vi "Update PhXP Parameters.vi"(8 "error in (no error)":errorcluster, 11 "VI in":refnum<vi>) -> (0 "error out":errorcluster, 2 "tau*":dbl[unit], 3 "f0":dbl[unit])   [LabVIEW 2019]
uses:
  Phasor Explorer Phasor Parameters.ctl
  Phasor Calculation Type.ctl
  SEPL Type.ctl
  Phasor Explorer Gate Parameters.ctl
  Gate Type.ctl
  SEPXP Gate Parameter to Adjust.ctl
  Phasor Explorer Decay Parameters.ctl
  IRF Model.ctl
  Phasor Explorer Display Parameters.ctl
  Type of Series.ctl
  Phasor Explorer Detector Parameters.ctl
panel:
  in  "Phasor Explorer Detector Parameters":T1={"Frames/Image"=0, "Gates/Frame"=1, "Bits/Frame"=1, "Multiplicity"=0, "Incident Signal"=0.0, "Poisson Signal"=FALSE} {"Frames/Image" min=1; "Multiplicity" min=0; "Bits/Frame" min=1; "Gates/Frame" min=1}
  in  "Edit User-defined Gate":bool
  in  "Phasor Explorer Display Parameters":T2={"# Points"=1, "Ramp Type"=enum."Linear", "Type of Series"=enum."1-Exp Decays", "Min tau"=0.0, "Max tau"=0.0, "Include 0"=FALSE, "Include Infinity"=FALSE} {"Min tau" min=0.0; "Max tau" min=0.0; "# Points" min=1 step=1}
  in  "Phasor Explorer Decay & IRF Parameters":T4 {"Lifetime" min=0.0; "IRF Period" min=0.0}
  in  "Gate Parameter to Adjust":T6 caption="Parameter to adjust"
  in  "Phasor Explorer Gate Parameters":T7={"First Gate Start"=0.0, "Use Gate Center"=FALSE, "Gate Width"=0.0, "Gate Step"=0.0, "# Gates"=1.0, "Gate Type"=enum."Square", "Edge Width"=0.0, "Top Slope"=0.0, "Reversed Sawtooth?"=FALSE, "Analytical Computation"=FALSE, "Integration"=enum."Item 0", "Tolerance"=1.0, "# Steps"=1.0, "Type of User-defined Function"=enum."Gate", "Use Gate Step"=FALSE} {"# Steps" min=0.0; "Tolerance" min=0.0; "Top Slope" min=0.0; "Edge Width" min=0.0; "Gate Step" min=0.0; "# Gates" min=1.0 step=1.0; "Gate Width" min=0.0}
  in  "Phasor Explorer Phasor Parameters":T9={"Harmonic frequency"=0.0, "Use f* = 1/D Frequency"=FALSE, "Calibrated Phasor"=FALSE, "Calibration Lifetime"=1e-09, "Phasor Calculation"=enum."Direct Sum", "SEPL Type"=enum."UC", "# Gates"=1.0, "Square Gate Width"=1e-09, "Show Ticks"=FALSE} {"Square Gate Width" min=0.0; "# Gates" min=0.0; "Calibration Lifetime" min=0.0; "Harmonic frequency" min=0.0}
  in  "Match Laser Period":bool
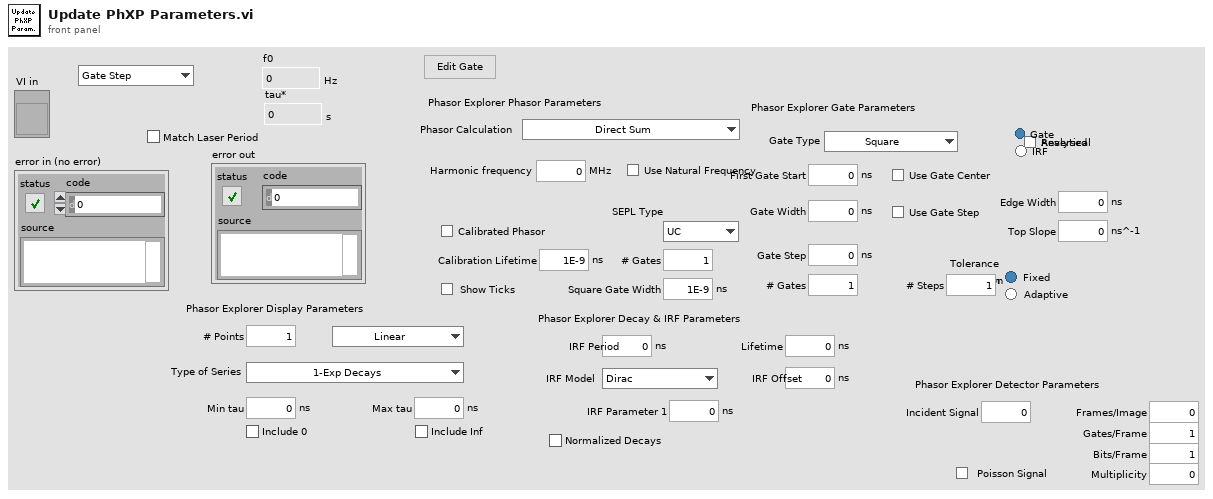
[diagram p1: front panel]
types:
  T1 = typedef "Phasor Explorer Detector Parameters.ctl" = cluster{"Frames/Image":i32, "Gates/Frame":i32, "Bits/Frame":i32, "Multiplicity":i32, "Incident Signal":dbl, "Poisson Signal":bool}
  T2 = typedef "Phasor Explorer Display Parameters.ctl" = cluster{"# Points":i32, "Ramp Type":enum16{"Linear", "Logarithmic"}, "Type of Series":T3, "Min tau":dbl[unit], "Max tau":dbl[unit], "Include 0":bool, "Include Infinity":bool}
  T3 = typedef "Type of Series.ctl" = enum16{"1-Exp Decays", "Linear Combination of 1-Exp"}
  T4 = typedef "Phasor Explorer Decay Parameters.ctl" = cluster{"Lifetime":dbl[unit], "IRF Offset":dbl[unit], "IRF Period":dbl[unit], "Normalized Decays":bool, "IRF Model":T5, "IRF Parameter 1":dbl[unit]}
  T5 = typedef "IRF Model.ctl" = enum16{"Dirac", "Exponential"}
  T6 = typedef "SEPXP Gate Parameter to Adjust.ctl" = enum16{"Gate Step", "# Gates"}
  T7 = typedef "Phasor Explorer Gate Parameters.ctl" = cluster{"First Gate Start":dbl[unit], "Use Gate Center":bool, "Gate Width":dbl[unit], "Gate Step":dbl[unit], "# Gates":dbl, "Gate Type":T8, "Edge Width":dbl[unit], "Top Slope":dbl[unit], "Reversed Sawtooth?":bool, "Analytical Computation":bool, "Integration":enum32{"Item 0", "Item 1"}, "Tolerance":dbl, "# Steps":dbl, "Type of User-defined Function":enum32{"Gate", "IRF"}, "Use Gate Step":bool}
  T8 = typedef "Gate Type.ctl" = enum16{"Square", "Finite Edge Square", "Finite Edge, Tilted Top Square", "Triangle", "Sawtooth", "User-defined"}
  T9 = typedef "Phasor Explorer Phasor Parameters.ctl" = cluster{"Harmonic frequency":dbl[unit], "Use f* = 1/D Frequency":bool, "Calibrated Phasor":bool, "Calibration Lifetime":dbl[unit], "Phasor Calculation":T10, "SEPL Type":T11, "# Gates":dbl, "Square Gate Width":dbl[unit], "Show Ticks":bool}
  T10 = typedef "Phasor Calculation Type.ctl" = enum16{"Direct Sum", "Analytical Formula"}
  T11 = typedef "SEPL Type.ctl" = enum16{"UC", "L_N", "L_N[W]"}
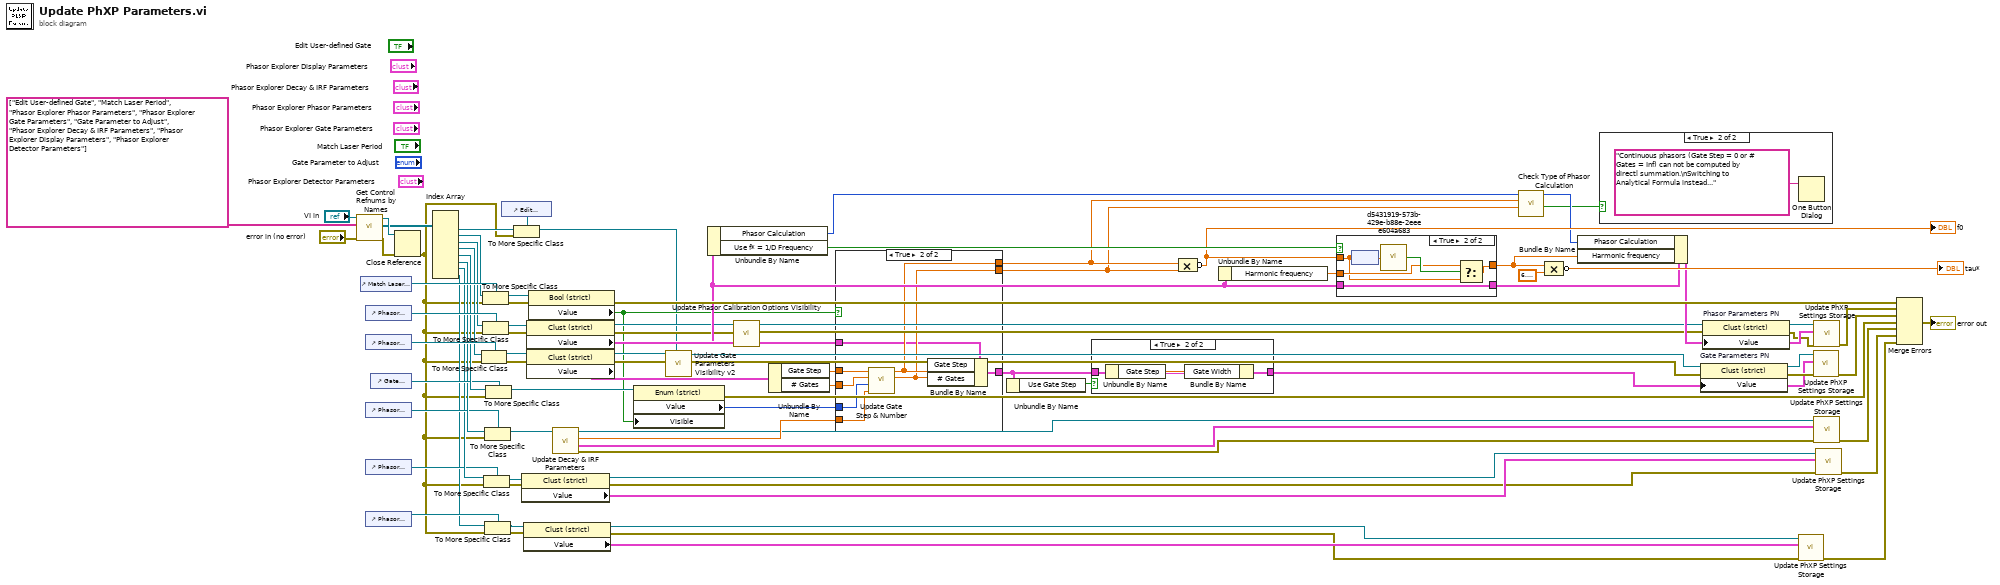
[diagram p0: block diagram]
diagram:
  n1 = call "Get Control Refnums by Names.vi"("error in"="error in (no error)", "Control Labels"=string[] ["Edit User-defined Gate", "Match Laser Period", "Phasor Explorer Phasor Parameters", "Phasor Explorer Gate Parameters", "Gate Parameter to Adjust", "Phasor Explorer Decay & IRF Parameters", "Phasor Explorer Display Parameters", "Phasor Explorer Detector Parameters"], "VI  Ref"="VI in") -> ("error out"=w18:errorcluster, "Ctl Refnums"=w84:refnum<vi>[], "VI  Ref (out)"=w85:refnum<vi>)  [unwired: 5 in, 1 out]
  n2 = control-ref of="Match Laser Period"() -> (w77:refnum<vi>)
  n3 = control-ref of="Phasor Explorer Phasor Parameters"() -> (w80:refnum<vi>)
  n4 = control-ref of="Phasor Explorer Gate Parameters"() -> (w79:refnum<vi>)
  n5 = control-ref of="Phasor Explorer Decay & IRF Parameters"() -> (w58:refnum<vi>)
  n6 = control-ref of="Phasor Explorer Display Parameters"() -> (w39:refnum<vi>)
  n7 = control-ref of="Phasor Explorer Detector Parameters"() -> (w14:refnum<vi>)
  n8 = control-ref of="Gate Parameter to Adjust"() -> (w71:refnum<vi>)
  n9 = Close Reference(reference=w85, error in (no error)=w18) -> (error out=w12:errorcluster)
  n10 = Index Array(array=w84) -> (element #1=w17:refnum<vi>, element #2=w62:refnum<vi>, element #3=w61:refnum<vi>, element #4=w60:refnum<vi>, element #5=w73:refnum<vi>, element #6=w59:refnum<vi>, element #7=w40:refnum<vi>, element #8=w13:refnum<vi>)  [unwired: 8 in]
  n11 = To More Specific Class(target class=w79, reference=w60, error in=w12) -> (specific class reference=w66:refnum<vi>, error out=w65:errorcluster)
  n12 = To More Specific Class(target class=w77, reference=w62, error in=w12) -> (specific class reference=w76:refnum<vi>, error out=w75:errorcluster)
  n13 = To More Specific Class(target class=w80, reference=w61, error in=w12) -> (specific class reference=w68:refnum<vi>, error out=w67:errorcluster)
  n14 = To More Specific Class(target class=w39, reference=w40, error in=w12) -> (specific class reference=w38:refnum<vi>, error out=w37:errorcluster)
  n15 = To More Specific Class(target class=w58, reference=w59, error in=w12) -> (specific class reference=w57:refnum<vi>)  [unwired: 1 out]
  n16 = To More Specific Class(target class=w14, reference=w13, error in=w12) -> (specific class reference=w11:refnum<vi>, error out=w10:errorcluster)
  n17 = To More Specific Class(target class=w71, reference=w73, error in=w12) -> (specific class reference=w72:refnum<vi>)  [unwired: 1 out]
  n18 = control-ref of="Edit User-defined Gate"() -> (w16:refnum<vi>)
  n19 = To More Specific Class(target class=w16, reference=w17, error in=w12) -> (specific class reference=w15:refnum<vi>)  [unwired: 1 out]
  n20 = property class="Clust (strict)"(reference=w38, error in=w37) -> (reference out=w34:refnum<vi>, error out=w32:errorcluster, "Value"=w33:T2)
  n21 = property class="Clust (strict)"(reference=w11, error in=w10) -> (reference out=w9:refnum<vi>, error out=w7:errorcluster, "Value"=w8:T1)
  n22 = property class="Clust (strict)"(reference=w68, error in=w67) -> (reference out=w26:refnum<vi>, error out=w24:errorcluster, "Value"=w47:T9)
  n23 = property class="Clust (strict)"(reference=w66, error in=w65) -> (reference out=w41:refnum<vi>, error out=w22:errorcluster, "Value"=w55:T7)
  n24 = property class="Bool (strict)"(reference=w76, error in=w75) -> (error out=w74:errorcluster, "Value"=w19:bool)  [unwired: 1 out]
  n25 = call "Update Decay & IRF Parameters.vi"("Decay & IRF Parameters Refnum"=w57) -> ("error out"=w29:errorcluster, "Value"=w31:T4, "Laser Period"=w56:dbl[unit], "Decay & IRF Parameters Refnum"=w30:refnum<vi>)  [unwired: 7 in]
  n26 = property class="Enum (strict)"(reference=w72, "Visible"=w19) -> (error out=w69:errorcluster, "Value"=w70:T6)  [unwired: 1 in, 1 out]
  n27 = call "Update Gate Parameters Visibility v2.vi"("Edit User-defined Gate"=w15, "error in (no error)"=w22, "Phasor Explorer Gate Parameters in"=w41) -> ("error out"=w21:errorcluster, "Phasor Explorer Gate Parameters out"=w20:refnum<vi>)  [unwired: 7 in]
  n28 = Unbundle By Name(w47) -> ("Phasor Calculation"=w28:T10, "Use f* = 1/D Frequency"=w83:bool)
  n29 = call "Update Phasor Calibration Options Visibility.vi"("Error In"=w24, "Phasor Explorer Phasor Parameters Refnum in"=w26) -> ("Error Out"=w23:errorcluster, "Phasor Explorer Phasor Parameters Refnum out"=w25:refnum<vi>)  [unwired: 8 in]
  n30 = Unbundle By Name(w55) -> ("Gate Step"=w64:dbl[unit], "# Gates"=w63:dbl)
  n31 = case shown="True" w19 {
    tunnel: w56 -> [_ w93]
    tunnel: [w91 w99] -> w53
    tunnel: [w90 w98] -> w52
    tunnel: w70 -> [_ w97]
    tunnel: w64 -> [w91 w96]
    tunnel: w63 -> [w90 w95]
    tunnel: w55 -> [w89 w94]
    tunnel: [w89 w92] -> w4
    frame False {
    }
    frame True {
      n32 = call "Update Gate Step & Number.vi"("Period"=w93, "Value to Update"=w97, "# Gates in"=w95, "Gate Step in"=w96) -> ("# Gates out"=w98:dbl, "Gate Step out"=w99:dbl[unit])  [unwired: 6 in]
      n33 = Bundle By Name(cluster=w94, "Gate Step"=w99, "# Gates"=w98) -> (w92:T7)
    }
  }
  n34 = Unbundle By Name(w4) -> ("Use Gate Step"=w5:bool)
  n35 = case shown="True" w5 {
    tunnel: w4 -> [w100 w102]
    tunnel: [w100 w101] -> w3
    frame False {
    }
    frame True {
      n36 = Unbundle By Name(w102) -> ("Gate Step"=w103:dbl[unit])
      n37 = Bundle By Name(cluster=w102, "Gate Width"=w103) -> (w101:T7)
    }
  }
  n38 = Compound Arithmetic op=MULTIPLY(w53, w52) -> (invert w48:dbl[unit])
  "f0" <- w48
  n39 = Unbundle By Name(w47) -> ("Harmonic frequency"=w46:dbl[unit])
  n40 = case shown="True" w83 {
    tunnel: w48 -> [_ w108]
    tunnel: [w104 w107] -> w2
    tunnel: w47 -> [w105 w111]
    tunnel: [w105 w111] -> w54
    tunnel: w46 -> [w104 w109]
    frame False {
    }
    frame True {
      # "update harmonic frequency"
      n41 = node(w108) -> (w106:dbl)
      n42 = call "d5431919-573b-429e-b88e-2eeee604a683.vi"("Number"=w106) -> ("Is NaN or Inf?"=w110:bool)  [unwired: 8 in]
      n43 = Select(t=w109, s=w110, f=w108) -> (s? t:f=w107:dbl[unit])
    }
  }
  n44 = call "Check Type of Phasor Calculation.vi"("# Gates"=w52, "Gate Step"=w53, "Phasor Calculation in"=w28) -> ("Changed?"=w1:bool, "Phasor Calculation out"=w27:T10)  [unwired: 7 in]
  n45 = Compound Arithmetic op=MULTIPLY(w2, 6.283185307179586) -> (invert →"tau*":dbl[unit])
  n46 = Bundle By Name(cluster=w54, "Phasor Calculation"=w27, "Harmonic frequency"=w2) -> (w49:T9)
  n47 = case shown="True" w1 {
    frame False {
    }
    frame True {
      n48 = One Button Dialog(message="Continuous phasors (Gate Step = 0 or # Gates = Inf) can not be computed by directl summation.\nSwitching to Analytical Formula instead...") -> ()  [unwired: 1 in, 1 out]
    }
  }
  n49 = property on="Gate Parameters PN" class="Clust (strict)"(reference=w20, error in=w21, "Value"=w3) -> (reference out=w43:refnum<vi>, error out=w42:errorcluster)
  n50 = property on="Phasor Parameters PN" class="Clust (strict)"(reference=w25, error in=w23, "Value"=w49) -> (reference out=w50:refnum<vi>, error out=w44:errorcluster)
  n51 = call "Update PhXP Settings Storage.vi"("Error In"=w7, "NewVal"=w8, "CtlRef"=w9) -> ("Error Out"=w6:errorcluster)  [unwired: 8 in]
  n52 = call "Update PhXP Settings Storage.vi"("Error In"=w42, "NewVal"=w3, "CtlRef"=w43) -> ("Error Out"=w45:errorcluster)  [unwired: 8 in]
  n53 = call "Update PhXP Settings Storage.vi"("Error In"=w44, "NewVal"=w49, "CtlRef"=w50) -> ("Error Out"=w51:errorcluster)  [unwired: 8 in]
  n54 = call "Update PhXP Settings Storage.vi"("Error In"=w29, "NewVal"=w31, "CtlRef"=w30) -> ("Error Out"=w36:errorcluster)  [unwired: 8 in]
  n55 = call "Update PhXP Settings Storage.vi"("Error In"=w32, "NewVal"=w33, "CtlRef"=w34) -> ("Error Out"=w35:errorcluster)  [unwired: 8 in]
  n56 = Merge Errors(w74, w51, w45, w69, w36, w35, w6) -> (→"error out":errorcluster)
